vi "test Deployment Disabled Custom Device.vi"(8 "error in":errorcluster, 11 "TestCase in":refnum<class "Deployment.lvclass">) -> (0 "error out":errorcluster, 3 "TestCase out":refnum<class "Deployment.lvclass">)   [LabVIEW 2020, in "Deployment.lvclass"]
uses:
  Deployment.lvclass
  <vilib>/addons/_JKI Toolkits/VI Tester/TestCase.llb/TestCase.lvclass
  315b1c3a-44c8-49e8-b756-01f865c29b4a.vi
  <vilib>/NI/VeriStand Custom Device Testing Tools/VeriStandTestUtilities/VeriStandTestUtilities.lvlib
  Scripting/AIM MIL-STD-1553 Scripting.lvlib
  C:/dev/git/niveristand-custom-device-testing-tools/VeriStandTestCase/VeriStandTestCase.lvclass
  C:/Program Files (x86)/National Instruments/LabVIEW 2020/vi.lib/addons/_JKI Toolkits/VI Tester/TestCase.llb/TestCase.lvclass
  C:/dev/git/niveristand-aim-milStd1553-custom-device/Source/Custom Device Support/Tests/System/Deployment/Deployment.lvclass
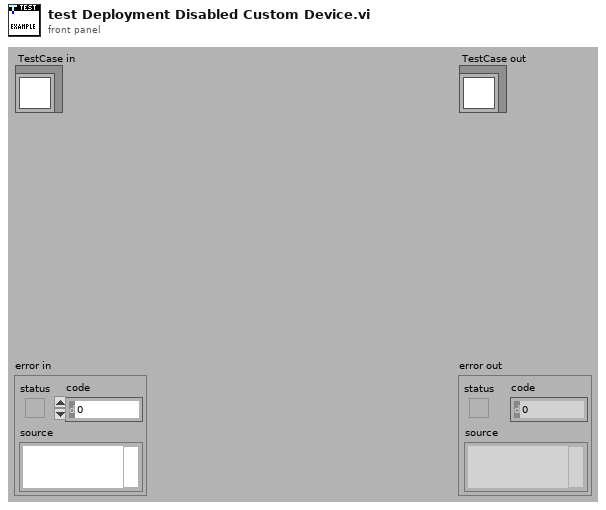
[diagram p1: front panel]
types:
  T1 = typedef "Custom Device API.lvlib/Custom Device Item Ref.ctl" = u64
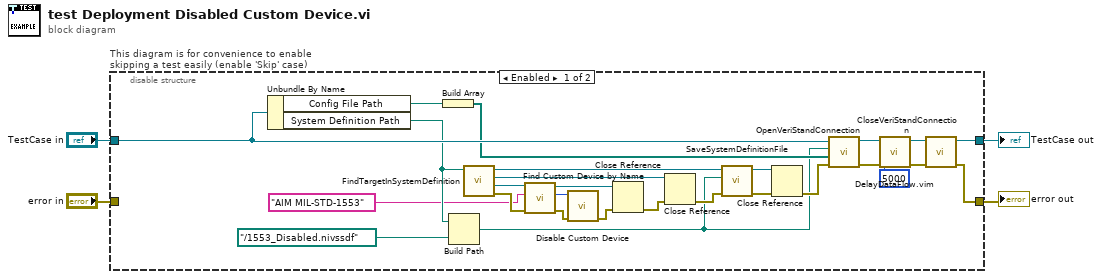
[diagram p0: block diagram]
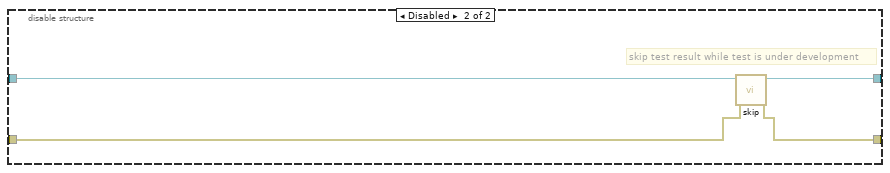
[diagram p2: hidden frame]
diagram:
  n1 = disable-structure "This diagram is for convenience to enable skipping a test easily (enable 'Skip' case)" shown="Enabled" {
    disable-tunnel: "TestCase in" -> [w24 w34]
    disable-tunnel: [w25 w32] -> w1
    disable-tunnel: [w27 w33] -> w3
    disable-tunnel: "error in" -> [_ w31]
    frame Enabled {
      n2 = Unbundle By Name(w24) -> ("Config File Path"=w22:path, "System Definition Path"=w14:path)
      n3 = Build Array(w22) -> (w21:path[])
      n4 = Build Path(base path=w14, name or relative path=path "../1553_Disabled.nivssdf") -> (appended path=w6:path)
      n5 = call <vilib>:"FindTargetInSystemDefinition.vi"("system definition path"=w14) -> ("error out"=w12:errorcluster, "Target"=w13:refnum<k24>, "Root"=w18:refnum<k24>, "System Definition"=w15:refnum<k24>)  [unwired: 7 in]
      n6 = call "Find Custom Device by Name.vi"("error in"=w12, "custom device name"="AIM MIL-STD-1553", "target"=w13) -> ("error out"=w10:errorcluster, "custom device"=w11:T1, "target out"=w8:refnum<k24>)  [unwired: 5 in, 1 out]
      n7 = call "Disable Custom Device.vi"("error in"=w10, "custom device ref"=w11) -> ("error out"=w9:errorcluster)  [unwired: 8 in, 1 out]
      n8 = Close Reference(reference=w8, error in (no error)=w9) -> (error out=w20:errorcluster)
      n9 = Close Reference(reference=w18, error in (no error)=w20) -> (error out=w19:errorcluster)
      n10 = call <vilib>:"SaveSystemDefinitionFile.vi"("error in (no error)"=w19, "System Definition File in"=w6, "System Definition Reference in"=w15) -> ("error out"=w17:errorcluster, "System Definition Reference out"=w16:refnum<k24>)  [unwired: 7 in]
      n11 = Close Reference(reference=w16, error in (no error)=w17) -> (error out=w7:errorcluster)
      n12 = call-dynamic "OpenVeriStandConnection.vi"("error in (no error)"=w7, "overrides files"=w21, "System Definition File"=w6, "VeriStand Test Case in"=w24) -> ("error out"=w30:errorcluster, "VeriStand Test Case out"=w26:refnum<class "Deployment.lvclass">)  [unwired: 5 in, 1 out]
      n13 = call "DelayDataFlow.vim"("value in"=w30, "milliseconds to wait"=u32 5000) -> ("value out"=w28:errorcluster)  [unwired: 2 in, 1 out]
      n14 = call-dynamic "CloseVeriStandConnection.vi"("error in (no error)"=w28, "VeriStand Test Case in"=w26) -> ("error out"=w27:errorcluster, "VeriStand Test Case out"=w25:refnum<class "Deployment.lvclass">)  [unwired: 8 in]
    }
    frame Disabled {
      # "skip test result while test is under development"
      n15 = call <vilib>:"skip.vi"("error in (no error)"=w31, "TestCase in"=w34) -> ("error out"=w33:errorcluster, "TestCase out"=w32:refnum<class "Deployment.lvclass">)  [unwired: 8 in]
    }
  }
  "error out" <- w3
  "TestCase out" <- w1
